vi "DrawARectangleCart.vi"(1 "height":i32, 2 "width":i32, 3 "y":i32, 4 "x":i32) -> (0 "picture":picture)   [LabVIEW 2010]
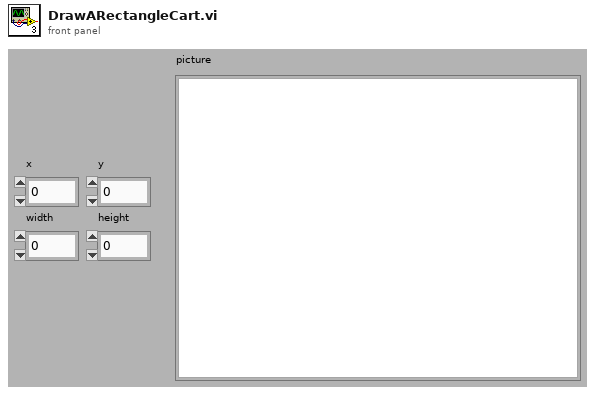
[diagram p1: front panel]
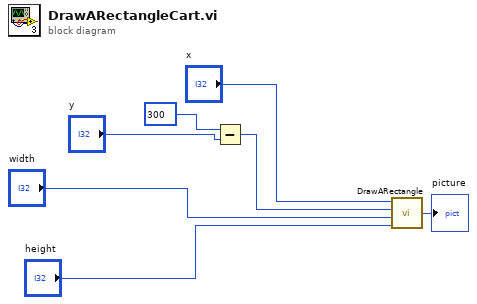
[diagram p0: block diagram]
diagram:
  n1 = Subtract(x=300, y="y") -> (x-y=w3:i32)
  n2 = call "DrawARectangle.vi"("height"="height", "width"="width", "y"=w3, "x"="x") -> ("picture"=→"picture":picture)
